vi "sor(SubVI).vi"(4 "Tolerancja":dbl, 6 "omega":dbl, 8 "Initial Guess":dbl[](array[numeric]), 10 "Macierz b":dbl[](array[numeric]), 11 "Macierz A":dbl[][](array[numeric])) -> (2 "Wykonana iczba Iteracji":i32, 3 "Metoda SOR":dbl[](array[numeric]))   [LabVIEW 2020]
uses:
  <vilib>/Analysis/Matrix/Numeric/Conversions/Array To Matrix - RA2.vi
  <vilib>/Analysis/Matrix/Numeric/Conversions/Array To Matrix - RA.vi
  <vilib>/addons/Multicore Analysis and Sparse Matrix/Linear Algebra/_linalg/Inverse Matrix (DBL).vi
  <vilib>/addons/Multicore Analysis and Sparse Matrix/BLAS/_blas/dgemm - General Matrix-Matrix Product (DBL).vi
  <vilib>/Analysis/Matrix/Numeric/Multiply/Multiply - RM,R.vi
  <vilib>/Analysis/BLAS.llb/dgemv - General Matrix-Vector Product (DBL).vi
  <vilib>/addons/Multicore Analysis and Sparse Matrix/BLAS/_blas/dgemv - General Matrix-Vector Product (DBL).vi
  <vilib>/Analysis/Matrix/NI_Matrix.lvlib
  <vilib>/Analysis/NI_AALBLAS.lvlib
  <vilib>/addons/Multicore Analysis and Sparse Matrix/BLAS/NI_MASM_BLAS.lvlib
  <vilib>/addons/Multicore Analysis and Sparse Matrix/Linear Algebra/NI_MASM_BasicLinAlg.lvlib
panel:
  out "Wczesny stop":bool
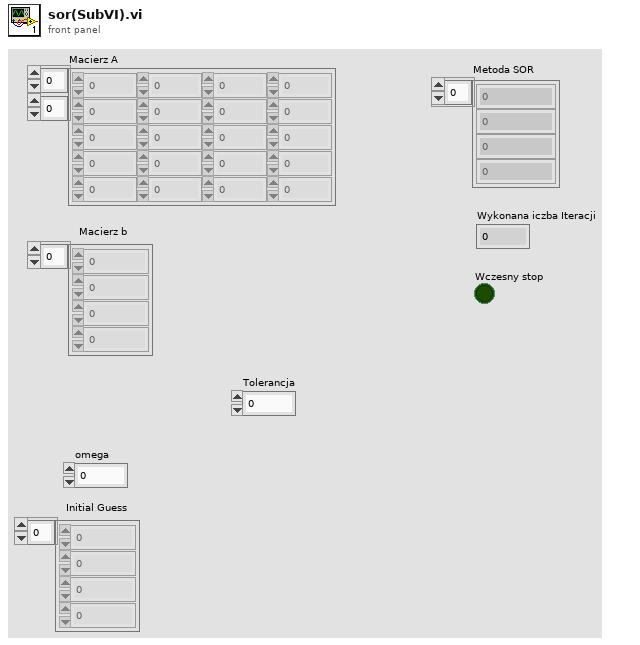
[diagram p1: front panel]
types:
  T1 = typedef "NI_Matrix.lvlib/RealMatrix.ctl" = dbl[][]
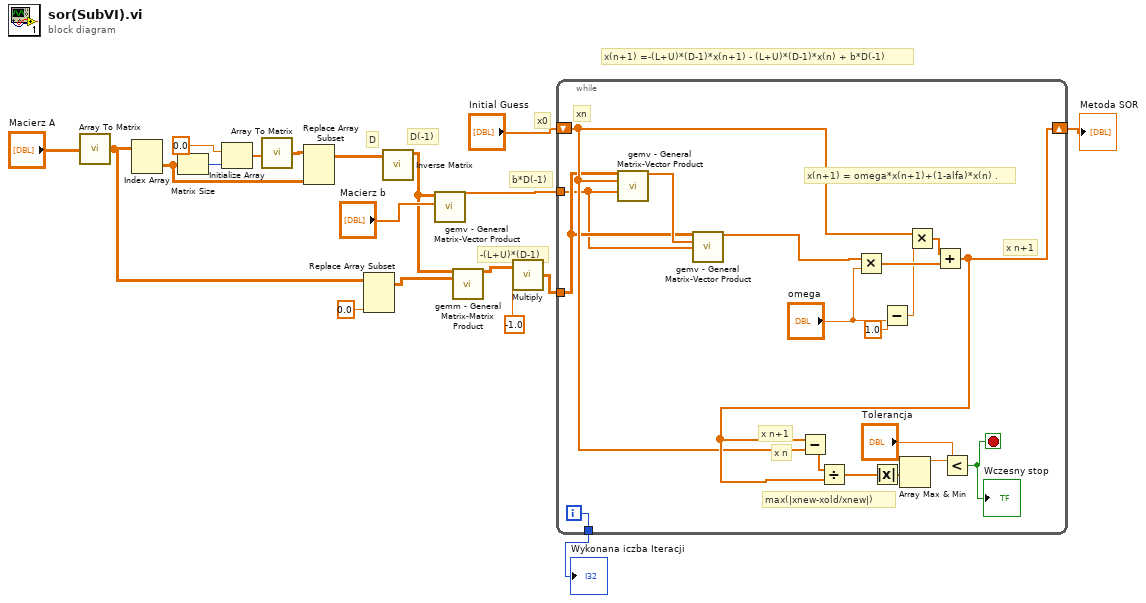
[diagram p0: block diagram]
diagram:
  # "x(n+1) =-(L+U)*(D-1)*x(n+1) - (L+U)*(D-1)*x(n) + b*D(-1)"
  # "b*D(-1)"
  # "-(L+U)*(D-1)"
  # "D(-1)"
  # "x0"
  # "D"
  n1 = call-poly <vilib>:"Array To Matrix.vi"("Real 2D Array"="Macierz A") -> ("Real Matrix"=w5:T1)
  n2 = Index Array(array=w5) -> (element=w9:T1)  [unwired: 2 in]
  n3 = Matrix Size(0:w9) -> (1:w13:i32)  [unwired: 1 out]
  n4 = Initialize Array(0.0 ("element"), w13) -> (w11:dbl[])
  n5 = call-poly <vilib>:"Array To Matrix.vi"("Real 1D Array"=w11) -> ("Real Matrix (Column Vector)"=w10:T1)
  n6 = Replace Array Subset(array=w10, new element=w9) -> (w7:T1)  [unwired: 2 in]
  n7 = Replace Array Subset(array=w5, new element=0.0 ("new diagonal/fill element")) -> (w2:T1)  [unwired: 2 in]
  n8 = call-poly <vilib>:"Inverse Matrix.vi"("Input Matrix"=w7) -> ("Inverse Matrix"=w3:T1)  [unwired: 9 in, 1 out]
  n9 = call-poly <vilib>:"gemv - General Matrix-Vector Product.vi"("x"="Macierz b", "A"=w3) -> ("dgemv"=w17:dbl[])  [unwired: 8 in, 1 out]
  n10 = call-poly <vilib>:"gemm - General Matrix-Matrix Product.vi"("A"=w3, "B"=w2) -> ("dgemm"=w1:T1)  [unwired: 12 in, 1 out]
  n11 = call-poly <vilib>:"Multiply.vi"("Real Scalar c"=-1.0 ("y"), "Real Matrix A"=w1) -> ("A * c"=w4:T1)
  n12 = while {
    tunnel: w17 -> [w22]
    shift-right: [w26] -> w6
    shift-left: "Initial Guess" -> [w25]
    tunnel: [w32] -> w15
    tunnel: w4 -> [w23]
    i -> [w32]
    stop <- w31 stop-if-true
    # "max(|xnew-xold/xnew|)"
    # "x n"
    # "x n+1"
    # "x(n+1) = omega*x(n+1)+(1-alfa)*x(n) ."
    # "xn"
    # "x n+1"
    n13 = call-poly <vilib>:"gemv - General Matrix-Vector Product.vi"("A"=w23, "x"=w25, "y"=w22) -> ("dgemv"=w24:dbl[])  [unwired: 11 in, 1 out]
    n14 = call-poly <vilib>:"gemv - General Matrix-Vector Product.vi"("A"=w23, "x"=w24, "y"=w22) -> ("dgemv"=w21:dbl[])  [unwired: 11 in, 1 out]
    n15 = Multiply(x=w21, y="omega") -> (x*y=w28:dbl[])
    n16 = Subtract(x=1.0, y="omega") -> (x-y=w27:dbl)
    n17 = Multiply(x=w25, y=w27) -> (x*y=w29:dbl[])
    n18 = Add(x=w29, y=w28) -> (x+y=w26:dbl[])
    n19 = Subtract(x=w26, y=w25) -> (x-y=w37:dbl[])
    n20 = Divide(x=w37, y=w26) -> (x/y=w36:dbl[])
    n21 = Absolute Value(x=w36) -> (abs(x)=w35:dbl[])
    n22 = Array Max & Min(array=w35) -> (max value=w34:dbl)  [unwired: 3 out]
    n23 = Less?(x=w34, y="Tolerancja") -> (x < y?=w31:bool)
    "Wczesny stop" <- w31
  }
  "Metoda SOR" <- w6
  "Wykonana iczba Iteracji" <- w15
